vi "lab2_sim_modem.vi"() -> ()   [LabVIEW 2014]
uses:
  <vilib>/addons/Modulation/Digital/General/MT Generate Bits (Galois, PN Order).vi
  <vilib>/addons/Modulation/Analog/support/mod_Set Error Source.vi
  <vilib>/addons/Modulation/Digital/Support/Common/Validators/mod_Generate Bits Validate.vi
  <vilib>/addons/Modulation/Digital/Support/Common/Validators/mod_AWGN Validate.vi
  <vilib>/addons/Modulation/Digital/Impairments/subVIs/mod_createSeeds.vi
  <vilib>/addons/Modulation/Digital/Support/Common/Validators/mod_Validate Samples Per Symbol.vi
  <vilib>/addons/Modulation/Analog/support/Validators/mod_Validate Complex Waveform.vi
  <vilib>/addons/Modulation/Analog/support/Validators/mod_WFErrorHandler.vi
  <vilib>/addons/Modulation/Digital/Support/Common/Validators/mod_Generate Filter Coefficients Validate.vi
  <vilib>/addons/Modulation/Digital/General/subVIs/mod_Generate Filter Coefficients.vi
  <vilib>/addons/Modulation/Digital/General/subVIs/mod_Generate Bits PN Sequence.vi
  <vilib>/addons/Modulation/Digital/General/MT Apply Pulse Shaping Filter (Generic).vi
  <vilib>/Analysis/1siggen.llb/Gaussian White Noise (obs 90).vi
  <vilib>/addons/Modulation/Digital/General/MT Apply Matched Filter (Generic).vi
  <vilib>/addons/Modulation/niDMT.lvlib
panel:
  out "received symbol":dbl
  out "error symbols":i32
  out "SER":dbl
  out "received bits":i32
  out "error bits":i32
  out "ber":dbl format="%#_5e"
  out "sync?":bool
  out "subarray":i16[](array[numeric])
  out "index map":u32[](array[numeric])
  out "output bit stream":i8[](array[numeric])
  in  "modulation":enum16{"PSK", "QAM"}(ring)
  in  "Gray code?":bool=TRUE
  out "size(s)":i32
  out "Received map":cdb[](graph)
  in  "Eb/N0 (10 dB)":dbl=10.0 format="%.2f"
  in  "samples per symbol":i32=16
  in  "filter parameter":dbl=0.5 format="%.2f"
  in  "filter length (symbols)":i32=8
  in  "pulse shaping filter (none)":T1(ring)=enum."Root Raised Cos"
  out "total bits":i32
  in  "total mod symbols":i32=2000 caption="total symbols"
  out "symbol map":cdb[](array[numeric])
  out "Transmitter map":cdb[](graph)
  in  "stop":bool
  in  "M-ARY":i32=4
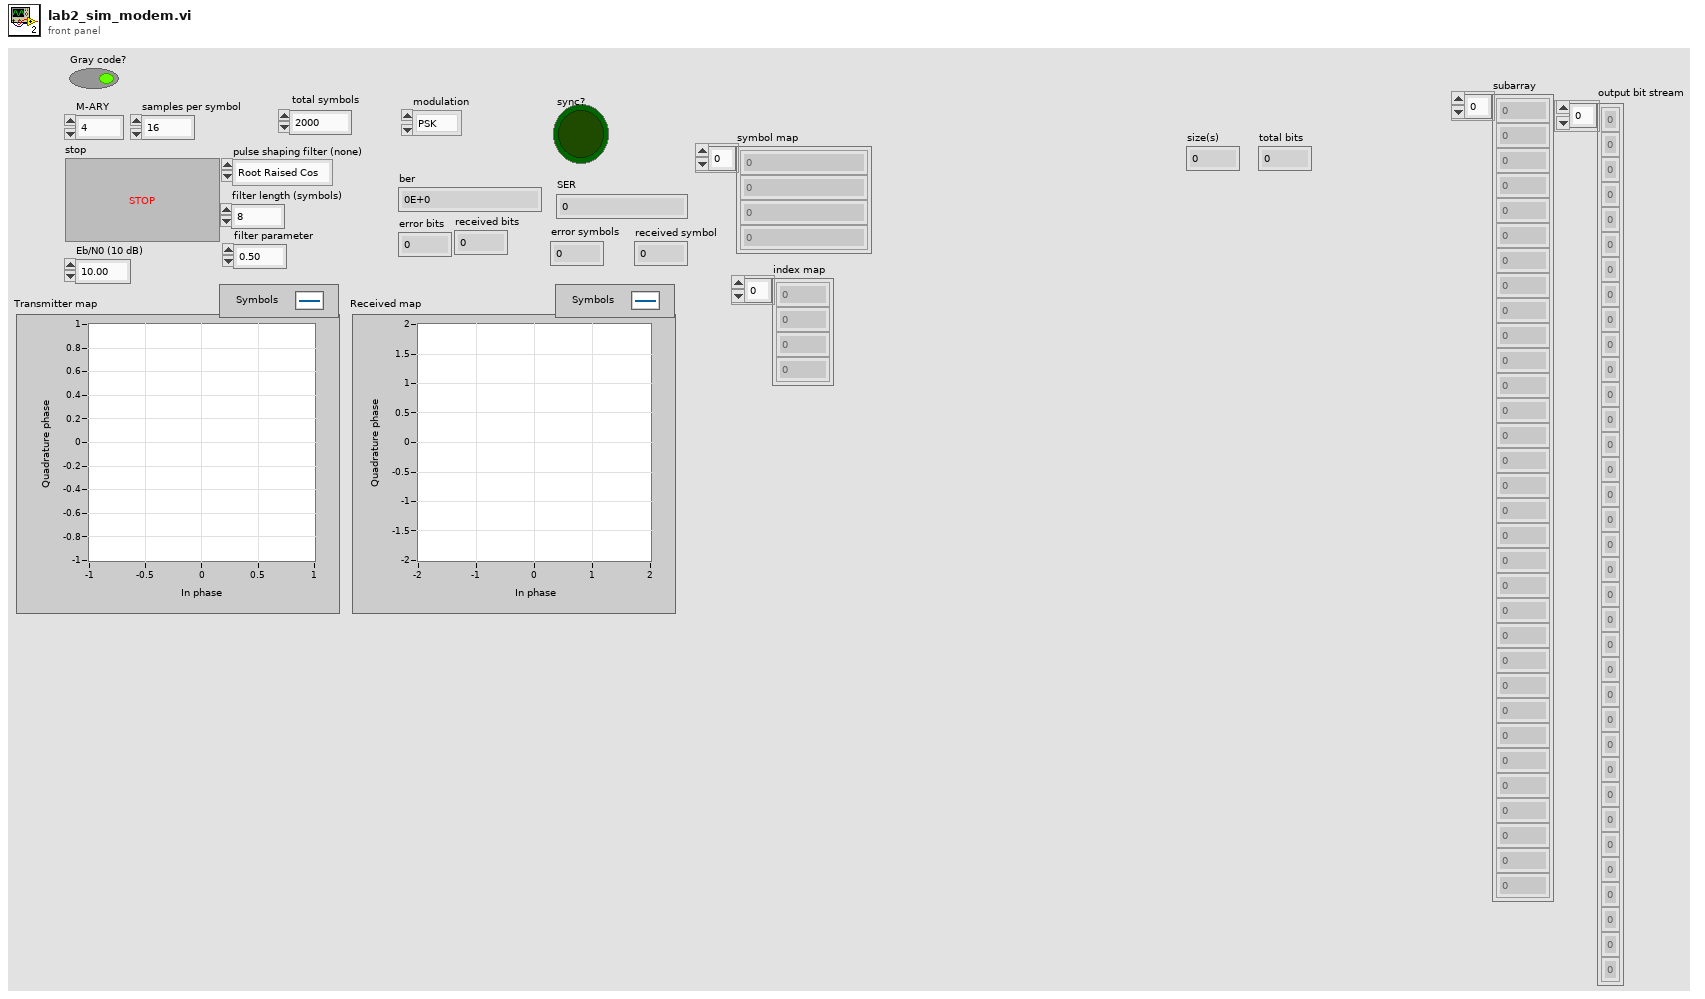
[diagram p1: front panel]
types:
  T1 = enum16{"none", "Raised Cosine", "Root Raised Cos", "Gaussian"}
  T2 = enum16{"FSK", "PSK", "QAM", "MSK", "PAM", "ASK", "CPM"}
  T3 = typedef "niAMT.lvlib/Complex Data Waveform.ctl" = cluster{"t0":dbl, "dt":dbl, "Y":cdb[]}
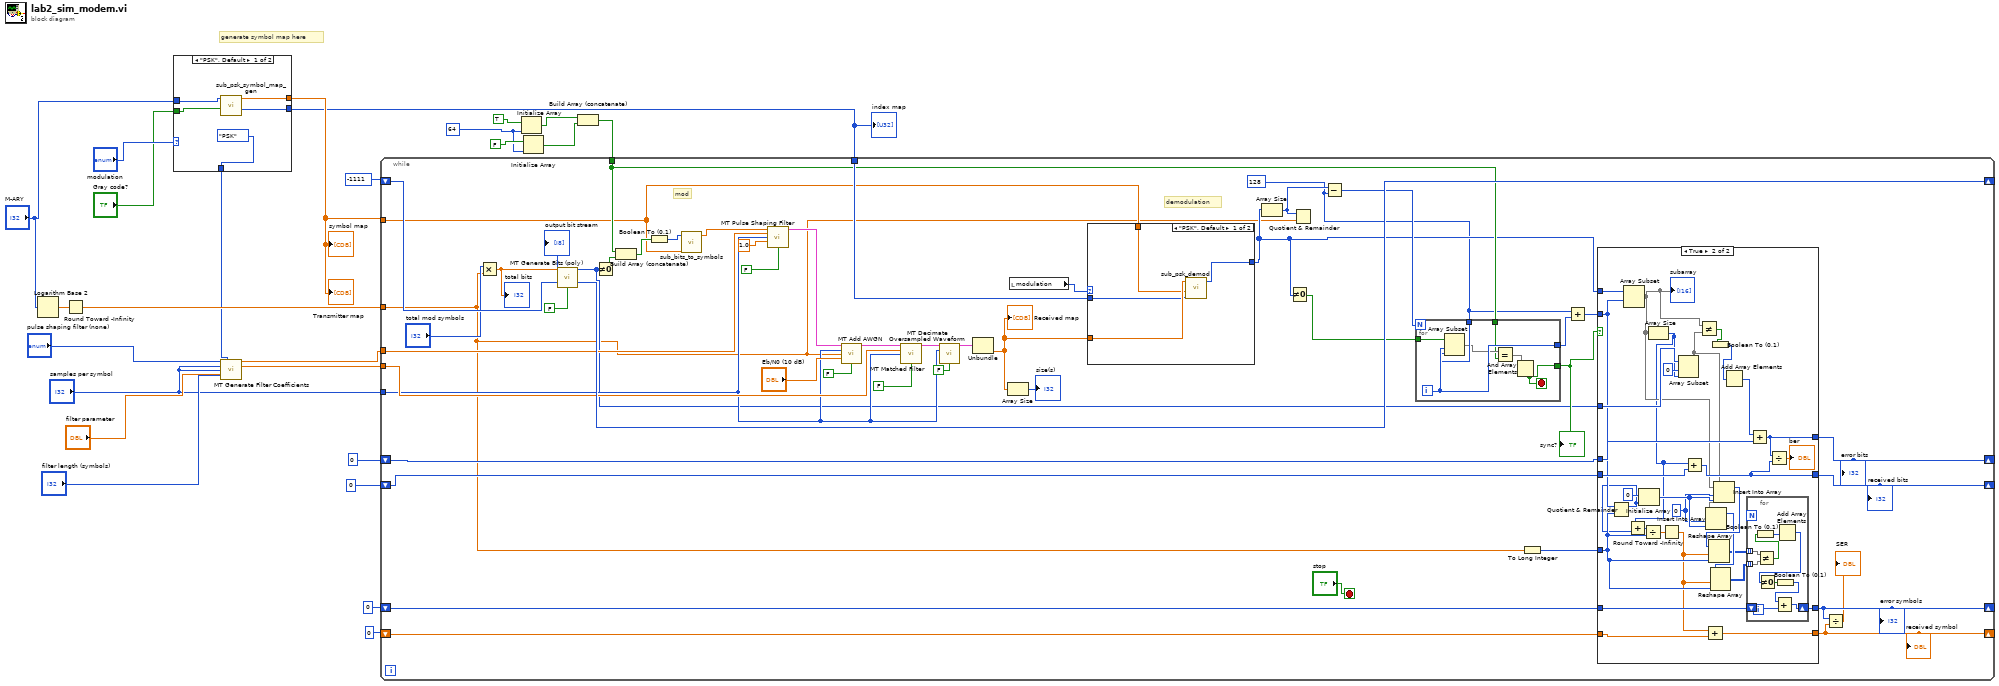
[diagram p0: block diagram]
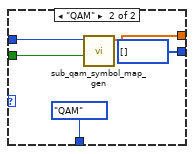
[diagram p2: hidden frame]
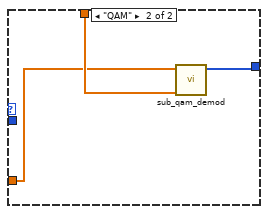
[diagram p4: hidden frame]
diagram:
  w5 = 64 ("dimension size")
  # "generate symbol map here"
  n1 = Logarithm Base 2(1:"M-ARY") -> (0:w25:dbl)
  n2 = Round Toward -Infinity(1:w25) -> (0:w18:dbl)
  n3 = case shown="\"PSK\", Default" "modulation" {
    tunnel: "M-ARY" -> [w29 w35]
    tunnel: "Gray code?" -> [w30 w34]
    tunnel: [w28 w33] -> w13
    tunnel: [T2."PSK" ("modulation type") T2."QAM" ("modulation type")] -> w12
    tunnel: [w26 u32[] [] ("index map")] -> w11
    frame "PSK", Default {
      n4 = call "sub_psk_symbol_map_gen.vi"("Gray code?"=w30, "M-PSK"=w29) -> ("index map"=w26:u32[], "symbol map"=w28:cdb[])  [unwired: 8 in]
    }
    frame "QAM" {
      n5 = call "sub_qam_symbol_map_gen.vi"("Gray code?"=w34, "M-QAM"=w35) -> ("symbol map"=w33:cdb[])  [unwired: 9 in]
    }
  }
  "Transmitter map" <- w13
  "symbol map" <- w13
  "index map" <- w11
  n6 = call <vilib>:"MT Generate Filter Coefficients.vi"("pulse shaping filter (none)"="pulse shaping filter (none)", "modulation type"=w12, "pulse shaping samples per symbol (16)"="samples per symbol", "matched samples per symbol (16)"="samples per symbol", "filter parameter"="filter parameter", "filter length (symbols)"="filter length (symbols)") -> ("pulse shaping filter coefficients"=w20:dbl[], "matched filter coefficients"=w17:dbl[])  [unwired: 7 in, 1 out]
  n7 = Initialize Array(TRUE, w5) -> (w10:bool[])
  n8 = Initialize Array(FALSE, w5) -> (w9:bool[])
  n9 = Build Array (concatenate)(w10, w9) -> (w6:bool[])
  n10 = while {
    tunnel: w13 -> [w44]
    shift-right: [w82] -> _
    shift-left: -1111 ("seed out") -> [w83]
    tunnel: w20 -> [w79]
    tunnel: "samples per symbol" -> [w69]
    tunnel: w18 -> [w42]
    tunnel: w17 -> [w71]
    tunnel: w11 -> [w64]
    tunnel: w6 -> [w59]
    shift-right: [w50] -> _
    shift-left: 0 -> [w51]
    shift-right: [w48] -> _
    shift-left: 0 -> [w49]
    shift-right: [w38] -> _
    shift-left: 0 -> [w40]
    shift-right: [w37] -> _
    shift-left: 0 -> [w39]
    stop <- "stop" stop-if-true
    w53 = 128
    # "demodulation"
    # "mod"
    n11 = Multiply(x="total mod symbols", y=w42) -> (x*y=w81:dbl)
    "total bits" <- w81
    n12 = call-poly <vilib>:"MT Generate Bits (poly).vi"("total bits (128)"=w81, "seed in (0xD6BF7DF2)"=w83, "reset? (T)"=FALSE) -> ("output bit stream"=w52:i8[], "seed out"=w82:i32)  [unwired: 10 in, 1 out]
    "output bit stream" <- w52
    n13 = Not Equal To 0?(x=w52) -> (x != 0?=w62:bool[])
    n14 = Build Array (concatenate)(w59, w62) -> (w46:bool[])
    n15 = Boolean To (0,1)(Boolean=w46) -> (0, 1=w45:i16[])
    n16 = call "sub_bits_to_symbols.vi"("symbol map"=w44, "bits"=w45) -> ("symbols"=w43:cdb[])  [unwired: 9 in]
    n17 = call-poly <vilib>:"MT Pulse Shaping Filter.vi"("symbols"=w43, "pulse shaping filter coefficients"=w79, "samples per symbol (16)"=w69, "symbol rate (Hz)"=1.0, "reset? (T)"=FALSE) -> ("output complex waveform"=w75:T3)  [unwired: 9 in, 1 out]
    n18 = call <vilib>:"MT Add AWGN.vi"("input complex waveform"=w75, "samples per symbol (16)"=w69, "bits per symbol (1)"=w42, "Eb/N0 (10 dB)"="Eb/N0 (10 dB)", "reset? (T)"=FALSE) -> ("output complex waveform"=w72:T3)  [unwired: 8 in, 2 out]
    n19 = call-poly <vilib>:"MT Matched Filter.vi"("input complex waveform"=w72, "matched filter coefficients"=w71, "samples per symbol (16)"=w69, "reset? (T)"=FALSE) -> ("output complex waveform"=w70:T3)  [unwired: 10 in, 1 out]
    n20 = call <vilib>:"MT Decimate Oversampled Waveform.vi"("input complex waveform"=w70, "decimation factor"=w69, "reset? (T)"=FALSE) -> ("output complex waveform"=w68:T3)  [unwired: 11 in, 1 out]
    n21 = Unbundle(w68) -> ("Y"=w65:cdb[])  [unwired: 2 out]
    "Received map" <- w65
    n22 = Array Size(array=w65) -> (size(s)=→"size(s)":i32)
    n23 = local read "modulation"() -> (w66:enum16{"PSK", "QAM"})
    n24 = case shown="\"PSK\", Default" w66 {
      tunnel: w65 -> [w139 w141]
      tunnel: w44 -> [w138 w142]
      tunnel: w64 -> [w137 _]
      tunnel: [w136 w140] -> w56
      frame "PSK", Default {
        n25 = call "sub_psk_demod.vi"("index map"=w137, "symbol map"=w138, "symbol"=w139) -> ("bitstream"=w136:i16[])  [unwired: 8 in]
      }
      frame "QAM" {
        n26 = call "sub_qam_demod.vi"("symbol map"=w142, "symbol"=w141) -> ("bitstream"=w140:i16[])  [unwired: 9 in]
      }
    }
    n27 = Array Size(array=w56) -> (size(s)=w61:i32)
    n28 = Not Equal To 0?(x=w56) -> (x != 0?=w57:bool[])
    n29 = Quotient & Remainder(x=w61, y=w42) -> ()  [unwired: 2 out]
    n30 = Subtract(x=w61, y=w53) -> (x-y=w60:i32)
    n31 = for {
      N: w60 -> [_]
      tunnel: w57 -> [w135]
      tunnel: [w134] -> w55
      tunnel: w53 -> [w133]
      tunnel: w59 -> [w131]
      tunnel: [w129] -> w58
      i -> [w134]
      stop <- w129 stop-if-true
      n32 = Array Subset(array=w135, index=w134, length=w133) -> (w132:bool[])
      n33 = Equal?(x=w132, y=w131) -> (x = y?=w130:bool[])
      n34 = And Array Elements(Boolean array=w130) -> (logical AND=w129:bool)
    }
    "sync?" <- w58
    n35 = To Long Integer(number=w42) -> (32bit integer=w41:i32)
    n36 = Add(x=w53, y=w55) -> (x+y=w54:i32)
    n37 = case shown="True" w58 {
      tunnel: w56 -> [_ w119]
      tunnel: w54 -> [_ w108]
      tunnel: w52 -> [_ w117]
      tunnel: w51 -> [w88 w114]
      tunnel: [w88 w112] -> w50
      tunnel: w49 -> [w87 w111]
      tunnel: [w87 w110] -> w48
      tunnel: w41 -> [_ w99]
      tunnel: [w86 w96] -> w38
      tunnel: w40 -> [w86 w95]
      tunnel: [w85 w94] -> w37
      tunnel: w39 -> [w85 w92]
      frame False {
      }
      frame True {
        w102 = 0
        n38 = Quotient & Remainder(x=w108, y=w99) -> (x-y*floor(x/y)=w91:i32)  [unwired: 1 out]
        n39 = Array Subset(array=w119, index=w108) -> (w105:i16[])  [unwired: 1 in]
        "subarray" <- w105
        n40 = Initialize Array(0, w91) -> (w103:i32[])
        n41 = Array Size(array=w105) -> (size(s)=w90:i32)
        n42 = Add(x=w90, y=w91) -> (x+y=w89:i32)
        n43 = Divide(x=w89, y=w99) -> (x/y=w106:dbl)
        n44 = Round Toward -Infinity(1:w106) -> (0:w93:dbl)
        n45 = Array Subset(array=w117, index=0, length=w90) -> (w104:i8[])
        n46 = Add(x=w90, y=w111) -> (x+y=w110:i32)
        n47 = Not Equal?(x=w105, y=w104) -> (x != y?=w116:bool[])
        n48 = Add(x=w93, y=w92) -> (x+y=w94:dbl)
        n49 = Insert Into Array(array=w104, index=w102, new element=w103) -> (w100:i8[])
        n50 = Boolean To (0,1)(Boolean=w116) -> (0, 1=w115:i16[])
        n51 = Reshape Array(w100, w93, w99) -> (w97:i8[][])
        n52 = Insert Into Array(array=w105, index=w102, new element=w103) -> (w101:i16[])
        n53 = Reshape Array(w101, w93, w99) -> (w98:i16[][])
        n54 = Add Array Elements(numeric array=w115) -> (sum=w113:i16)
        n55 = for {
          tunnel: w98 -> [w127] mode=indexing
          tunnel: w97 -> [w128] mode=indexing
          shift-right: [w121] -> w96
          shift-left: w95 -> [w120]
          n56 = Not Equal?(x=w127, y=w128) -> (x != y?=w126:bool[])
          n57 = Boolean To (0,1)(Boolean=w126) -> (0, 1=w125:i16[])
          n58 = Add Array Elements(numeric array=w125) -> (sum=w124:i16)
          n59 = Not Equal To 0?(x=w124) -> (x != 0?=w123:bool)
          n60 = Boolean To (0,1)(Boolean=w123) -> (0, 1=w122:i16)
          n61 = Add(x=w122, y=w120) -> (x+y=w121:i32)
        }
        n62 = Add(x=w113, y=w114) -> (x+y=w112:i32)
        n63 = Divide(x=w112, y=w110) -> (x/y=→"ber":dbl)
      }
    }
    "error bits" <- w50
    "received bits" <- w48
    "error symbols" <- w38
    "received symbol" <- w37
    n64 = Divide(x=w38, y=w37) -> (x/y=→"SER":dbl)
  }
